vi "CreateActionMessage.vi"(2 "Value":i32, 3 "Key":u32, 4 "Action":u8=1, 5 "Device":u8=1) -> (1 "Message":string)   [LabVIEW 2021]
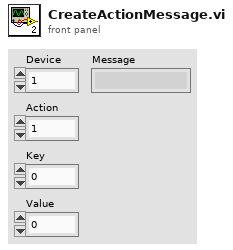
[diagram p1: front panel]
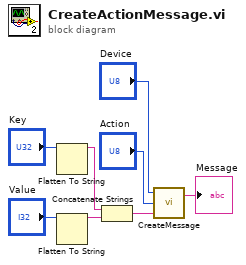
[diagram p0: block diagram]
diagram:
  n1 = Flatten To String(anything="Key") -> (data string=w7:string)  [unwired: 3 in, 2 out]
  n2 = Flatten To String(anything="Value") -> (data string=w6:string)  [unwired: 3 in, 2 out]
  n3 = Concatenate Strings(w7, w6) -> (w5:string)
  n4 = call "CreateMessage.vi"("Payload"=w5, "Operation"="Action", "Device"="Device") -> ("Message"=→"Message":string)  [unwired: 1 in]
